vi "FindReceiver.vi"(8 "error in (no error)":errorcluster, 10 "Game":refnum<class "Game.lvclass">, 11 "object in":refnum<class "DefendGoalTactic.lvclass">) -> (0 "error out":errorcluster, 1 "Dist":dbl, 2 "Receiver Id":i32, 3 "object out":refnum<class "DefendGoalTactic.lvclass">)   [LabVIEW 2024, in "DefendGoalTactic.lvclass"]
uses:
  DefendGoalTactic.lvclass
  Game_class/Game.lvclass
  Game_class/Game.lvclass/Game.ctl
  Parameters_class/Parameters.lvclass/Parameters.ctl
  Team_class/Team.lvclass/Team.ctl
  Object_class/Object.lvclass/Object.ctl
  Ball_class/Ball.lvclass/Ball.ctl
  Robot_class/Robot.lvclass/Robot.ctl
  <vilib>/Analysis/coordinate.llb/2D Cartesian Coordinate Shift (Scalar).vi
  <vilib>/Analysis/coordinate.llb/2D Cartesian Coordinate Rotation (Scalar).vi
  Robot_class/Read id.vi
  Object_class/Read position(x,y).vi
  Game_class/Read Parameters.lvclass.vi
  Game_class/Read EnemyRef.vi
  Game_class/Read BallRef.vi
  Game_class/Read NewParameters.vi
  Game_class/Read OffensiveTeam.vi
  Team_class/Read RobotRef.vi
  Ball_class/Read v_x.vi
  Ball_class/Read v_y.vi
  Parameters_class/Read AttakingOurselves.vi
  Ally_class/Ally.lvclass
  C:/Users/ROBOIME2/Documents/SSL ROBOIME/SSL_AI/Team_class/Team.lvclass
  Ball_class/Ball.lvclass
  C:/Users/ROBOIME2/Documents/SSL ROBOIME/SSL_AI/Object_class/Object.lvclass
  Enemy_class/Enemy.lvclass
  Robot_class/Robot.lvclass
  Parameters_class/Parameters.lvclass
  <vilib>/Analysis/NI_AALPro.lvlib
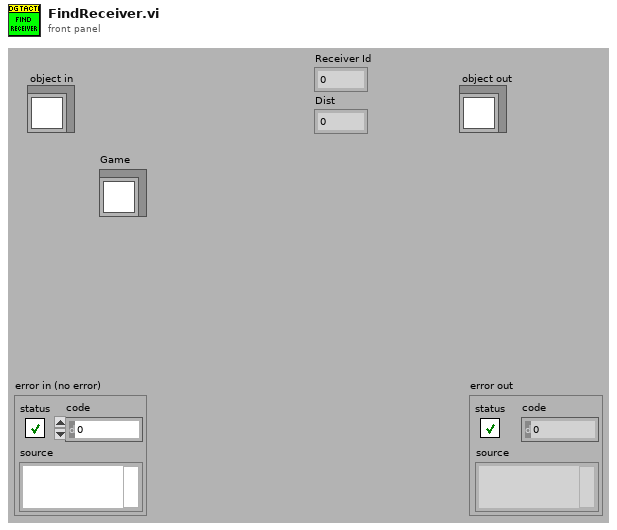
[diagram p1: front panel]
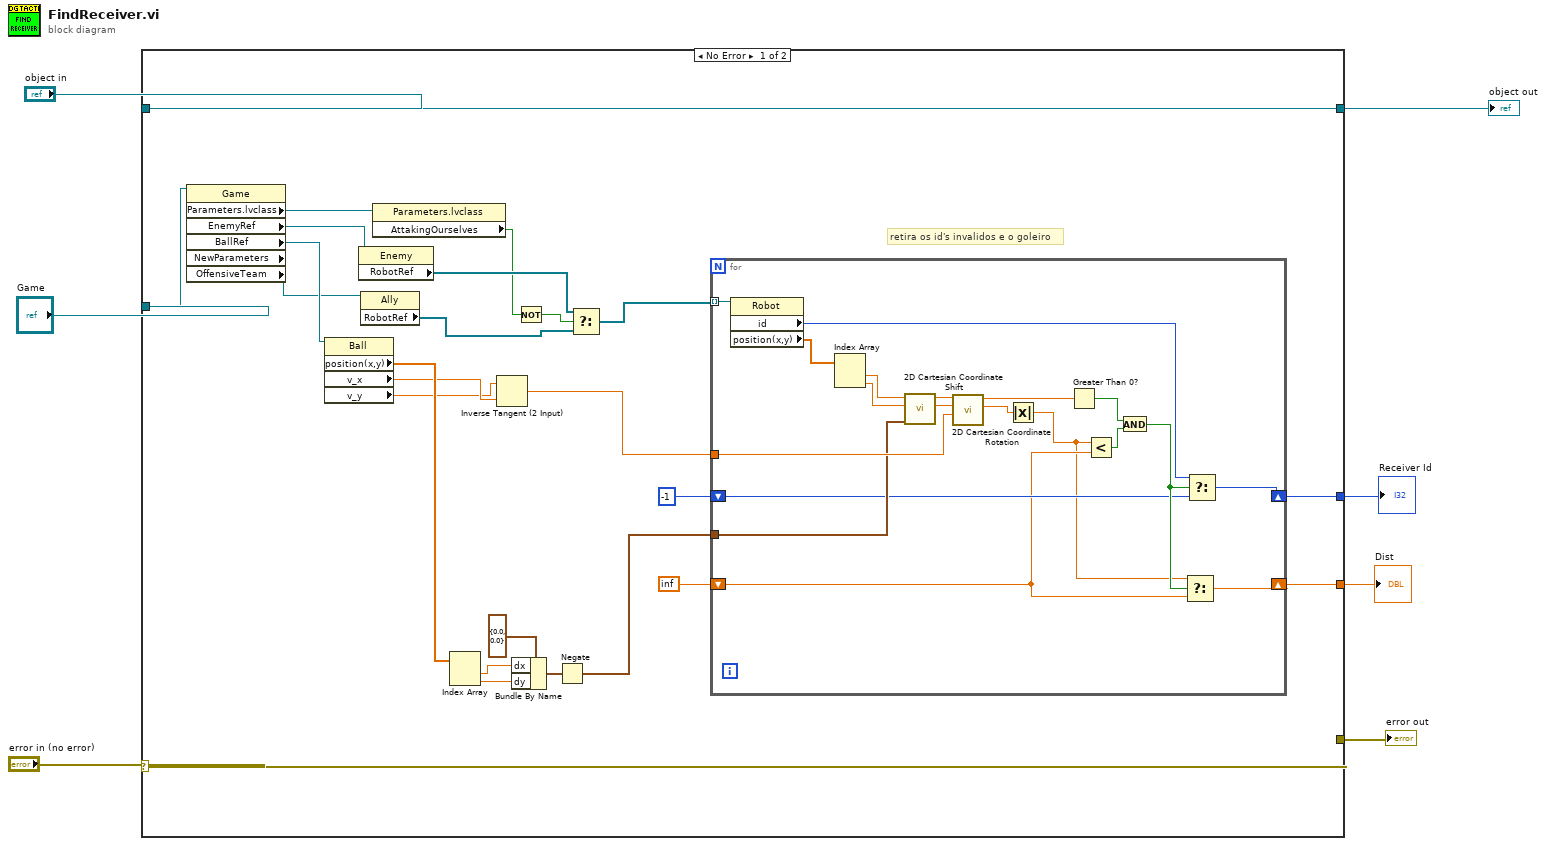
[diagram p0: block diagram]
diagram:
  n1 = case shown="No Error" "error in (no error)" {
    selector: "error in (no error)" -> [w31 w53]
    tunnel: [w31 w53] -> w6
    tunnel: [w32 w52] -> w4
    tunnel: "object in" -> [w32 w52]
    tunnel: "Game" -> [w20 _]
    tunnel: [w9 _] -> w2
    tunnel: [w8 _] -> w1
    frame No Error {
      # "retira os id's invalidos e o goleiro"
      n2 = property class="Game" props=["Parameters.lvclass", "EnemyRef", "BallRef", "NewParameters", "OffensiveTeam"](reference=w20) -> ("Parameters.lvclass"=w19:refnum<class "Parameters.lvclass">, "EnemyRef"=w30:refnum<class "Enemy.lvclass">, "BallRef"=w29:refnum<class "Ball.lvclass">, "OffensiveTeam"=w22:refnum<class "Ally.lvclass">)  [unwired: 1 in, 3 out]
      n3 = property class="Ball"(reference=w29) -> ("position(x,y)"=w12:dbl[], "v_x"=w11:dbl, "v_y"=w10:dbl)  [unwired: 1 in, 2 out]
      n4 = property class="Enemy"(reference=w30) -> ("RobotRef"=w24:refnum<class "Robot.lvclass">[])  [unwired: 1 in, 2 out]
      n5 = property class="Ally"(reference=w22) -> ("RobotRef"=w21:refnum<class "Robot.lvclass">[])  [unwired: 1 in, 2 out]
      n6 = property class="Parameters.lvclass"(reference=w19) -> ("AttakingOurselves"=w18:bool)  [unwired: 1 in, 2 out]
      n7 = Index Array(array=w12) -> (element #1=w14:dbl, element #2=w13:dbl)  [unwired: 2 in]
      n8 = Inverse Tangent (2 Input)(1:w11, 2:w10) -> (0:w28:dbl)
      n9 = Bundle By Name(cluster=cluster{"dx":dbl, "dy":dbl} {"dx"=0.0, "dy"=0.0} ("shift"), "dx"=w14, "dy"=w13) -> (w26:cluster{"dx":dbl, "dy":dbl})
      n10 = Not(x=w18) -> (.not. x?=w17:bool)
      n11 = Negate(x=w26) -> (-x=w25:cluster{"dx":dbl, "dy":dbl})
      n12 = Select(t=w24, s=w17, f=w21) -> (s? t:f=w23:refnum<class "Robot.lvclass">[])
      n13 = for {
        tunnel: w23 -> [w51] mode=indexing
        tunnel: w28 -> [w50]
        tunnel: w25 -> [w48]
        shift-right: [w37] -> w9
        shift-left: -1 -> [w38]
        shift-right: [w36] -> w8
        shift-left: inf -> [w35]
        n14 = property class="Robot"(reference=w51) -> ("id"=w39:i32, "position(x,y)"=w49:dbl[])  [unwired: 1 in, 2 out]
        n15 = Index Array(array=w49) -> (element #1=w47:dbl, element #2=w46:dbl)  [unwired: 2 in]
        n16 = call-poly <vilib>:"2D Cartesian Coordinate Shift.vi"("shift"=w48, "y"=w46, "x"=w47) -> ("y out"=w44:dbl, "x out"=w45:dbl)  [unwired: 6 in, 1 out]
        n17 = call-poly <vilib>:"2D Cartesian Coordinate Rotation.vi"("theta"=w50, "y"=w44, "x"=w45) -> ("y out"=w34:dbl, "x out"=w42:dbl)  [unwired: 6 in, 1 out]
        n18 = Absolute Value(x=w34) -> (abs(x)=w33:dbl)
        n19 = Greater Than 0?(x=w42) -> (x > 0?=w43:bool)
        n20 = Less?(x=w33, y=w35) -> (x < y?=w41:bool)
        n21 = And(x=w43, y=w41) -> (x .and. y?=w40:bool)
        n22 = Select(t=w33, s=w40, f=w35) -> (s? t:f=w36:dbl)
        n23 = Select(t=w39, s=w40, f=w38) -> (s? t:f=w37:i32)
      }
    }
    frame Error {
    }
  }
  "error out" <- w6
  "object out" <- w4
  "Receiver Id" <- w2
  "Dist" <- w1
